vi "mat2txt.vi"(1 "file path 2":path caption="文件路径 （空时为对话框）") -> (0 "Unique Temporary File Path":path)   [LabVIEW 2014]
panel:
  out "standard output":string caption="标准输出"
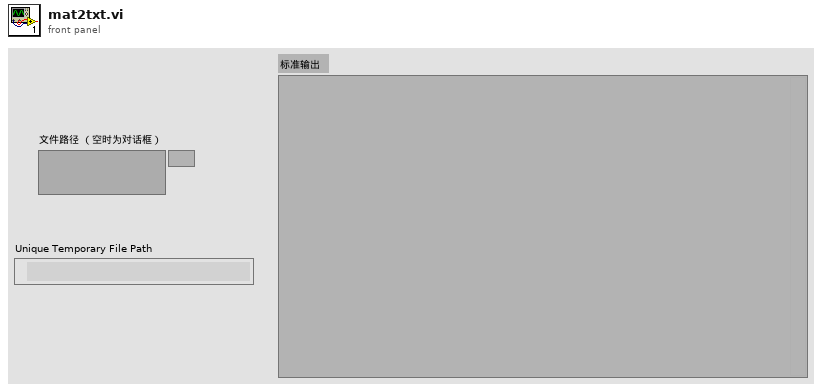
[diagram p1: front panel]
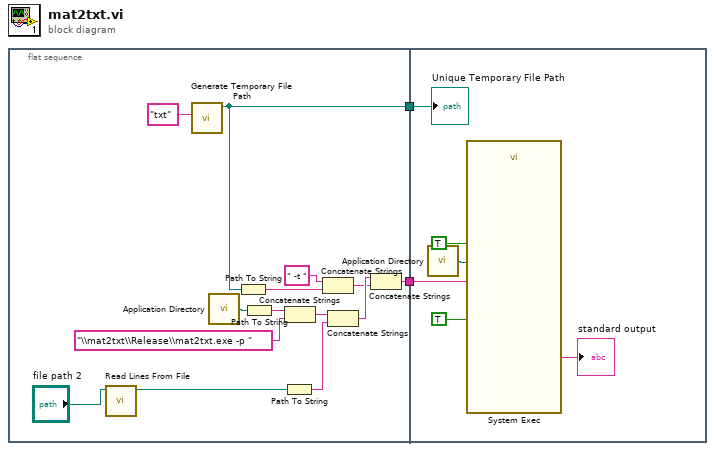
[diagram p0: block diagram]
diagram:
  n1 = flat-sequence {
    tunnel: [w16] -> w2
    tunnel: [w15] -> w1
    tunnel: w2 -> [w18]
    tunnel: w1 -> [w19]
    frame #0 {
      n2 = call <vilib>:"Read Lines From File.vi"("file path (dialog if empty)"="file path 2") -> ("new file path (Not A Path if cancelled)"=w13:path)  [unwired: 5 in, 3 out]
      n3 = call <vilib>:"Generate Temporary File Path.vi"("Temporary File Extension (tmp)"="txt") -> ("Unique Temporary File Path"=w15:path)  [unwired: 9 in, 1 out]
      n4 = call <vilib>:"Application Directory.vi"() -> ("Application Directory"=w5:path)
      n5 = Path To String(path=w15) -> (string=w4:string)
      n6 = Path To String(path=w5) -> (string=w7:string)
      n7 = Path To String(path=w13) -> (string=w12:string)
      n8 = Concatenate Strings(w7, "\\mat2txt\\Release\\mat2txt.exe -p ") -> (w6:string)
      n9 = Concatenate Strings(" -t ", w4) -> (w10:string)
      n10 = Concatenate Strings(w6, w12) -> (w11:string)
      n11 = Concatenate Strings(w11, w10) -> (w16:string)
    }
    frame #1 {
      n12 = call <vilib>:"Application Directory.vi"() -> ("Application Directory"=w17:path)
      n13 = call <vilib>:"System Exec.vi"("run minimized? (F)"=TRUE, "wait until completion? (T)"=TRUE, "working directory"=w17, "command line"=w18) -> ("standard output"=→"standard output":string)  [unwired: 4 in, 3 out]
      "Unique Temporary File Path" <- w19
    }
  }
